vi "Query_Scope_Response.vi"() -> ()   [LabVIEW 2025]
panel:
  out "read buffer":string
  in  "write buffer":string
  in  "VISA resource name":refnum<visa-resource-name>
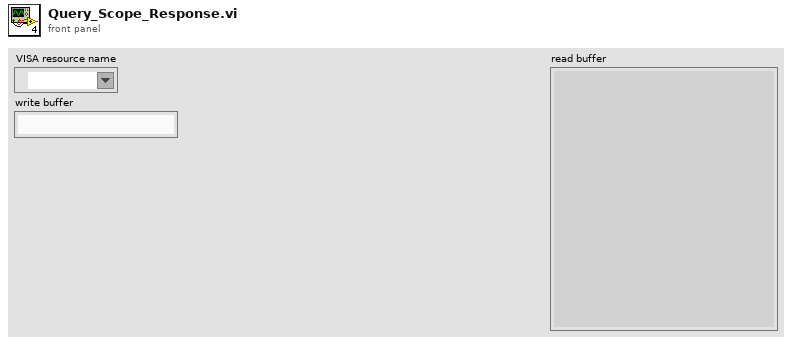
[diagram p1: front panel]
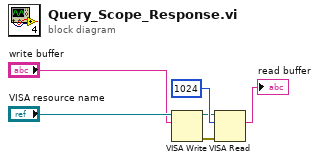
[diagram p0: block diagram]
diagram:
  n1 = VISA Write(VISA resource name="VISA resource name", write buffer="write buffer") -> (VISA resource name out=w1:refnum<visa-resource-name>, error out=w2:errorcluster)  [unwired: 1 in, 1 out]
  n2 = VISA Read(VISA resource name=w1, byte count=u32 1024, error in (no error)=w2) -> (read buffer=→"read buffer":string)  [unwired: 3 out]
